vi "Save Data Workspace Info.vi"() -> (0 "Workspace Info":T1={"Device Name"="test", "Device Info"="test", "Path"=path "C:/Users/gio/Desktop/test"})   [LabVIEW 2014]
uses:
  SaveData Workspace Info.ctl
panel:
  # "LICENSED MATERIALS – PROPERTY OF IBM\nCopyright IBM Corp. 2016,\nALL RIGHTS RESERVED"
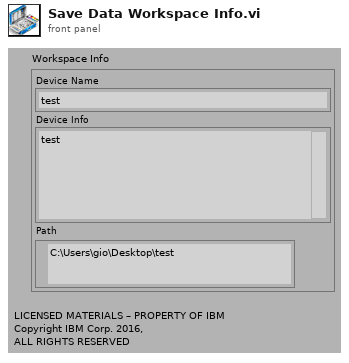
[diagram p1: front panel]
types:
  T1 = typedef "SaveData Workspace Info.ctl" = cluster{"Device Name":string, "Device Info":string, "Path":path}
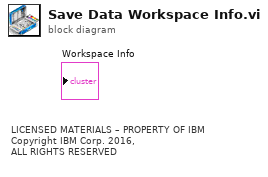
[diagram p0: block diagram]
diagram:
  # "LICENSED MATERIALS – PROPERTY OF IBM\nCopyright IBM Corp. 2016,\nALL RIGHTS RESERVED"
